vi "Run Bfr Tx - Handle Transmit Size.vi"(5 "Buffer Size":u64, 7 "Buffer Option":T1, 8 "error in (no error)":errorcluster, 11 "Transmit Bytes":T2) -> (0 "error out":errorcluster, 2 "Bytes to Transmit":i32, 3 "Transmit?":bool)   [LabVIEW 2019, in "UDP-Custom-Device Engine.lvlib"]
uses:
  UDP-Custom-Device Engine.lvlib
  <vilib>/NI/NIVS Inline Async API/_Data Access Engine/Data Access Engine/Types/Read.DVR.ctl
  <vilib>/NI/NIVS Inline Async API/_Data Access Engine/Access Type Classes/Read/Read.lvclass
  Shared/Types/Shared - Transmit Buffer Options.ctl
  <vilib>/NI/NIVS Inline Async API/_Data Access Engine/Access Type Classes/Read/Read.lvclass/Read.ctl
  <vilib>/NI/NIVS Inline Async API/_Data Access Engine/Data Access Engine/Methods/Read.Data.vi
  <vilib>/NI VeriStand/VeriStand Data/Type Conversion/Type Conversion.From Double (I32).vi
  <vilib>/NI/NIVS Inline Async API/_Data Access Engine/Access Type Classes/Read/Read.ProcessData.vi
  <vilib>/NI VeriStand/VeriStand Data/VeriStand Data.lvlib
  <vilib>/NI/NIVS Inline Async API/_Data Access Engine/Data Access Engine/Data Access Engine.lvclass
  Shared/UDP-Custom-Device Shared.lvlib
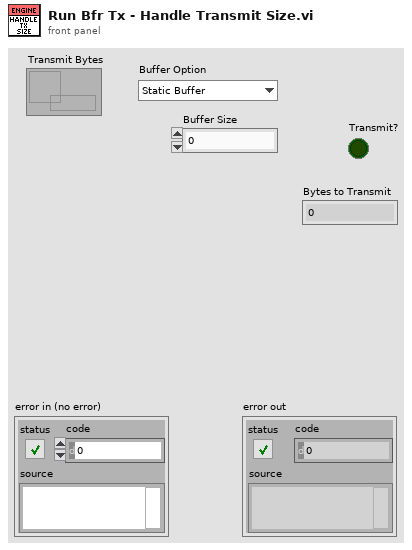
[diagram p1: front panel]
types:
  T1 = typedef "UDP-Custom-Device Shared.lvlib/Shared - Transmit Buffer Options.ctl" = enum16{"Static Buffer", "FIFO Buffer", "FIFO Buffer + Port"}
  T2 = typedef "Data Access Engine.lvlib/Data Access Engine.lvclass/Read.DVR.ctl" = refnum<data-value>
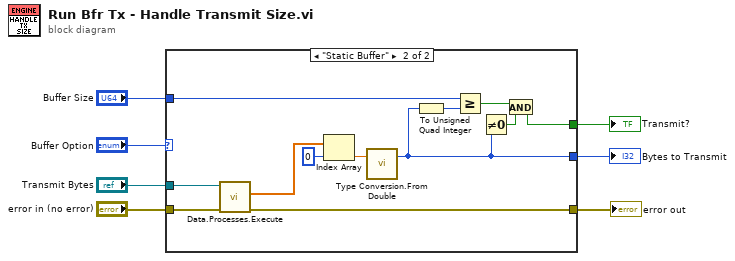
[diagram p0: block diagram]
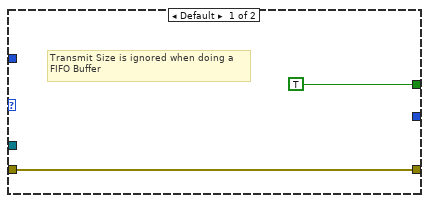
[diagram p2: hidden frame]
diagram:
  n1 = case shown="\"Static Buffer\"" "Buffer Option" {
    tunnel: "Transmit Bytes" -> [_ w19]
    tunnel: "error in (no error)" -> [w8 w18]
    tunnel: [w8 w17] -> w5
    tunnel: [_ w14] -> w4
    tunnel: [TRUE w11] -> w3
    tunnel: "Buffer Size" -> [_ w15]
    frame Default {
      # "Transmit Size is ignored when doing a\nFIFO Buffer"
    }
    frame "Static Buffer" {
      n2 = call-poly <vilib>:"Data.Processes.Execute.vi"("error in (no error)"=w18, "Ref"=w19) -> ("error out"=w17:errorcluster, "Values"=w21:dbl[])  [unwired: 7 in, 1 out]
      n3 = Index Array(array=w21, index=0) -> (element=w16:dbl)
      n4 = call-poly <vilib>:"Type Conversion.From Double.vi"("value in"=w16) -> ("value out"=w14:i32)  [unwired: 2 in]
      n5 = To Unsigned Quad Integer(1:w14) -> (0:w10:u64)
      n6 = Greater Or Equal?(x=w15, y=w10) -> (x >= y?=w13:bool)
      n7 = Not Equal To 0?(x=w14) -> (x != 0?=w12:bool)
      n8 = And(x=w13, y=w12) -> (x .and. y?=w11:bool)
    }
  }
  "error out" <- w5
  "Transmit?" <- w3
  "Bytes to Transmit" <- w4
